vi "Read Conditional Channels.vi"(8 "error in (no error)":errorcluster, 11 "Output Sequencer in":refnum<class "Output Sequencer.lvclass">) -> (0 "error out":errorcluster, 3 "Output Sequencer out":refnum<class "Output Sequencer.lvclass">)   [LabVIEW 2024, in "Output Sequencer.lvlib" / "Output Sequencer.lvclass"]
uses:
  Output Sequencer.lvclass
  Output Sequencer.lvclass/Output Sequencer.ctl
  <vilib>/FlexLogger/SDK/PluginSDK.lvlibp/PEFClasses/SDK/Plugin/Plugin.lvclass
  C:/Program Files/National Instruments/LabVIEW 2024/vi.lib/FlexLogger/SDK/PluginSDK.lvlibp/PEFClasses/SDK/Plugin/Plugin.lvclass
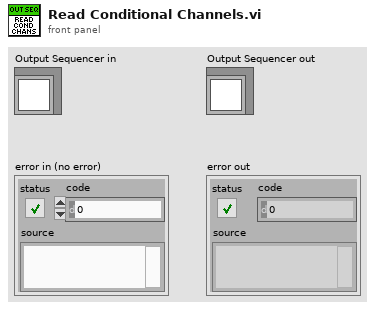
[diagram p1: front panel]
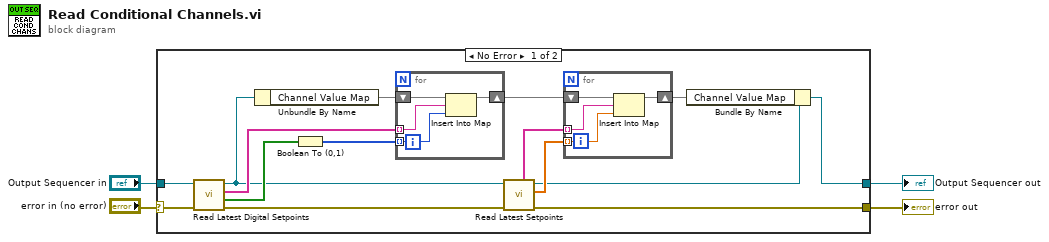
[diagram p0: block diagram]
diagram:
  n1 = case shown="No Error" "error in (no error)" {
    selector: "error in (no error)" -> [w5 w28]
    tunnel: [w14 w29] -> w4
    tunnel: [w13 w28] -> w3
    tunnel: "Output Sequencer in" -> [w12 w29]
    frame No Error {
      n2 = call <vilib>:"Read Latest Digital Setpoints.vi"("error in (no error)"=w5, "Plugin in"=w12) -> ("error out"=w19:errorcluster, "Values"=w16:bool[], "Names"=w15:string[], "Plugin out"=w8:refnum<class "Output Sequencer.lvclass">)  [unwired: 6 in]
      n3 = Unbundle By Name(w8) -> ("Channel Value Map"=w11:map{string, dbl})
      n4 = Boolean To (0,1)(Boolean=w16) -> (0, 1=w10:i16[])
      n5 = for {
        shift-right: [w26] -> w7
        shift-left: w11 -> [w27]
        tunnel: w15 -> [w25] mode=indexing
        tunnel: w10 -> [w24] mode=indexing
        n6 = Insert Into Map(map in=w27, key=w25, value=w24) -> (map out=w26:map{string, dbl})  [unwired: 2 out]
      }
      n7 = call <vilib>:"Read Latest Setpoints.vi"("error in (no error)"=w19, "Plugin in"=w8) -> ("error out"=w13:errorcluster, "Channel Setpoints"=w17:dbl[], "Plugin out"=w6:refnum<class "Output Sequencer.lvclass">, "Names"=w18:string[])  [unwired: 6 in]
      n8 = for {
        shift-right: [w22] -> w9
        shift-left: w7 -> [w23]
        tunnel: w18 -> [w21] mode=indexing
        tunnel: w17 -> [w20] mode=indexing
        n9 = Insert Into Map(map in=w23, key=w21, value=w20) -> (map out=w22:map{string, dbl})  [unwired: 2 out]
      }
      n10 = Bundle By Name(cluster=w6, "Channel Value Map"=w9) -> (w14:refnum<class "Output Sequencer.lvclass">)
    }
    frame Error {
    }
  }
  "Output Sequencer out" <- w4
  "error out" <- w3
